vi "GUI_StagingCameras.vi"() -> ()   [LabVIEW 2013]
uses:
  shared programs/GUI_Template/GUI_master/tcp_new_data_event.ctl
  shared programs/GUI_Template/GUI_master/tcp new data cluster.ctl
  <vilib>/vision/Image Controls.llb/IMAQ Image.ctl
panel:
  in  "Target.X::9":dbl=200.0 caption="Target X" format="%#.2p"
  in  "Target.Y::9":dbl=200.0 caption="Target Y" format="%#.2p"
  in  "Target.X::8":dbl=200.0 caption="Target X" format="%#.2p"
  in  "Target.Y::8":dbl=200.0 caption="Target Y" format="%#.2p"
  in  "Target.X::7":dbl=200.0 caption="Target X" format="%#.2p"
  in  "Target.Y::7":dbl=200.0 caption="Target Y" format="%#.2p"
  in  "Target.X::6":dbl=200.0 caption="Target X" format="%#.2p"
  in  "Target.Y::6":dbl=200.0 caption="Target Y" format="%#.2p"
  in  "Target.X::5":dbl=200.0 caption="Target X" format="%#.2p"
  in  "Target.Y::5":dbl=200.0 caption="Target Y" format="%#.2p"
  in  "Target.X::4":dbl=200.0 caption="Target X" format="%#.2p"
  in  "Target.Y::4":dbl=200.0 caption="Target Y" format="%#.2p"
  in  "Target.X::3":dbl=200.0 caption="Target X" format="%#.2p"
  in  "Target.Y::3":dbl=200.0 caption="Target Y" format="%#.2p"
  in  "Target.X::2":dbl=200.0 caption="Target X" format="%#.2p"
  in  "Target.Y::2":dbl=200.0 caption="Target Y" format="%#.2p"
  in  "Target.Y::1":dbl=200.0 caption="Target Y" format="%#.2p"
  in  "Target.X::1":dbl=200.0 caption="Target X" format="%#.2p"
  in  "MaxGUIPixel::9":dbl=200.0 caption="Max GUI pixel" format="%#.2p"
  in  "MaxGUIPixel::8":dbl=200.0 caption="Max GUI pixel" format="%#.2p"
  in  "MaxGUIPixel::7":dbl=200.0 caption="Max GUI pixel" format="%#.2p"
  in  "MaxGUIPixel::6":dbl=200.0 caption="Max GUI pixel" format="%#.2p"
  in  "MaxGUIPixel::5":dbl=200.0 caption="Max GUI pixel" format="%#.2p"
  in  "MaxGUIPixel::4":dbl=200.0 caption="Max GUI pixel" format="%#.2p"
  in  "MaxGUIPixel::3":dbl=200.0 caption="Max GUI pixel" format="%#.2p"
  in  "MaxGUIPixel::2":dbl=200.0 caption="Max GUI pixel" format="%#.2p"
  in  "MaxGUIPixel::1":dbl=200.0 caption="Max GUI pixel" format="%#.2p"
  in  "Position.Axis 1::13":dbl=0.001 caption="x" step=0.003 format="%.3f"
  in  "Position.Axis 2::13":dbl=0.001 caption="y" step=0.003 format="%.3f"
  in  "Position.Axis 3::13":dbl=0.001 caption="x" step=0.001 format="%.3f"
  in  "Position.Axis 4::13":dbl=0.001 caption="y" step=0.001 format="%.3f"
  in  "GUIdevice 13":string="TREX TRA1"
  in  "Position.Axis 1::12":dbl=0.001 caption="x" step=0.003 format="%.3f"
  in  "GUIdevice 12":string="StagingTRA3"
  in  "Position.Axis 2::12":dbl=0.001 caption="y" step=0.003 format="%.3f"
  in  "Position.Axis 1::11":dbl=0.001 caption="x" step=0.003 format="%.3f"
  in  "GUIdevice 11":string="StagingTRA2"
  in  "Position.Axis 2::11":dbl=0.001 caption="y" step=0.003 format="%.3f"
  in  "Position.Axis 3::11":dbl=0.001 caption="x" step=0.0001 format="%.3f"
  in  "Position.Axis 4::11":dbl=0.001 caption="y" step=0.001 format="%.3f"
  in  "Position.Axis 5::11":dbl=0.001 caption="x" step=0.003 format="%.3f"
  in  "Position.Axis 6::11":dbl=0.001 caption="y" step=0.003 format="%.3f"
  in  "Position.Axis 6::10":dbl=0.001 caption="y" step=0.003 format="%.3f"
  in  "Position.Axis 5::10":dbl=0.001 caption="x" format="%.3f"
  in  "Position.Axis 4::10":dbl=0.001 caption="y" step=0.003 format="%.3f"
  in  "Position.Axis 3::10":dbl=0.001 caption="x" step=0.003 format="%.3f"
  in  "Position.Axis 2::10":dbl=0.001 caption="y" step=0.003 format="%.3f"
  in  "GUIdevice 10":string="StagingTRA1"
  in  "Position.Axis 1::10":dbl=0.001 caption="x" step=0.003 format="%#.3p"
  out "image::2":T1(plugin-control) caption="StagingM1Far"
  in  "exposure::2":dbl=0.001 caption="exposure" format="%#.2p"
  in  "exposure::3":dbl=0.001 caption="exposure" format="%#.2p"
  out "image::3":T1(plugin-control) caption="StagingOAP2Near"
  in  "exposure::1":dbl=0.001 caption="exposure" format="%#.2p"
  out "image::1":T1(plugin-control) caption="StagingM1Near"
  in  "GUIdevice 9":string="StagingAlignBeam2"
  in  "exposure::9":dbl=0.001 caption="exposure" format="%#.2p"
  out "image::9":T1(plugin-control) caption="StagingAlignBeam2"
  in  "exposure::8":dbl=0.001 caption="exposure" format="%#.2p"
  out "image::8":T1(plugin-control) caption="StagingOAP2Far"
  in  "exposure::7":dbl=0.001 caption="exposure" format="%#.2p"
  out "image::7":T1(plugin-control) caption="StagingOAP1Far"
  in  "GUIdevice 8":string="StagingOAP2Far"
  in  "GUIdevice 7":string="StagingOAP1Far"
  in  "GUIdevice 6":string="StagingAlignBeam1"
  in  "exposure::6":dbl=0.001 caption="exposure" format="%#.2p"
  out "image::6":T1(plugin-control) caption="StagingAlignBeam1"
  in  "exposure::5":dbl=0.001 caption="exposure" format="%#.2p"
  out "image::5":T1(plugin-control) caption="StagingOAP1Near"
  in  "exposure::4":dbl=0.001 caption="exposure" format="%#.2p"
  out "image::4":T1(plugin-control) caption="StagingM3Far"
  in  "GUIdevice 5":string="StagingOAP1Near"
  in  "GUIdevice 4":string="StagingM3Far"
  in  "GUIdevice 3":string="StagingOAP2Near"
  in  "GUIdevice 2":string="StagingM1Far"
  out "error IO 2":errorcluster
  out "tcp data event":T2
  in  "GUIdevice 1":string="StagingM1Near"
  in  "insert tag":bool=TRUE
  in  "stop":bool
  # "STAGING CAMERAS"
  # "M20"
  # "SW Mirror"
  # "M1"
  # "M3"
  # "OAP1 Mirror"
  # "BS mirror"
  # "OAP 2"
  # "M5"
  # "M4"
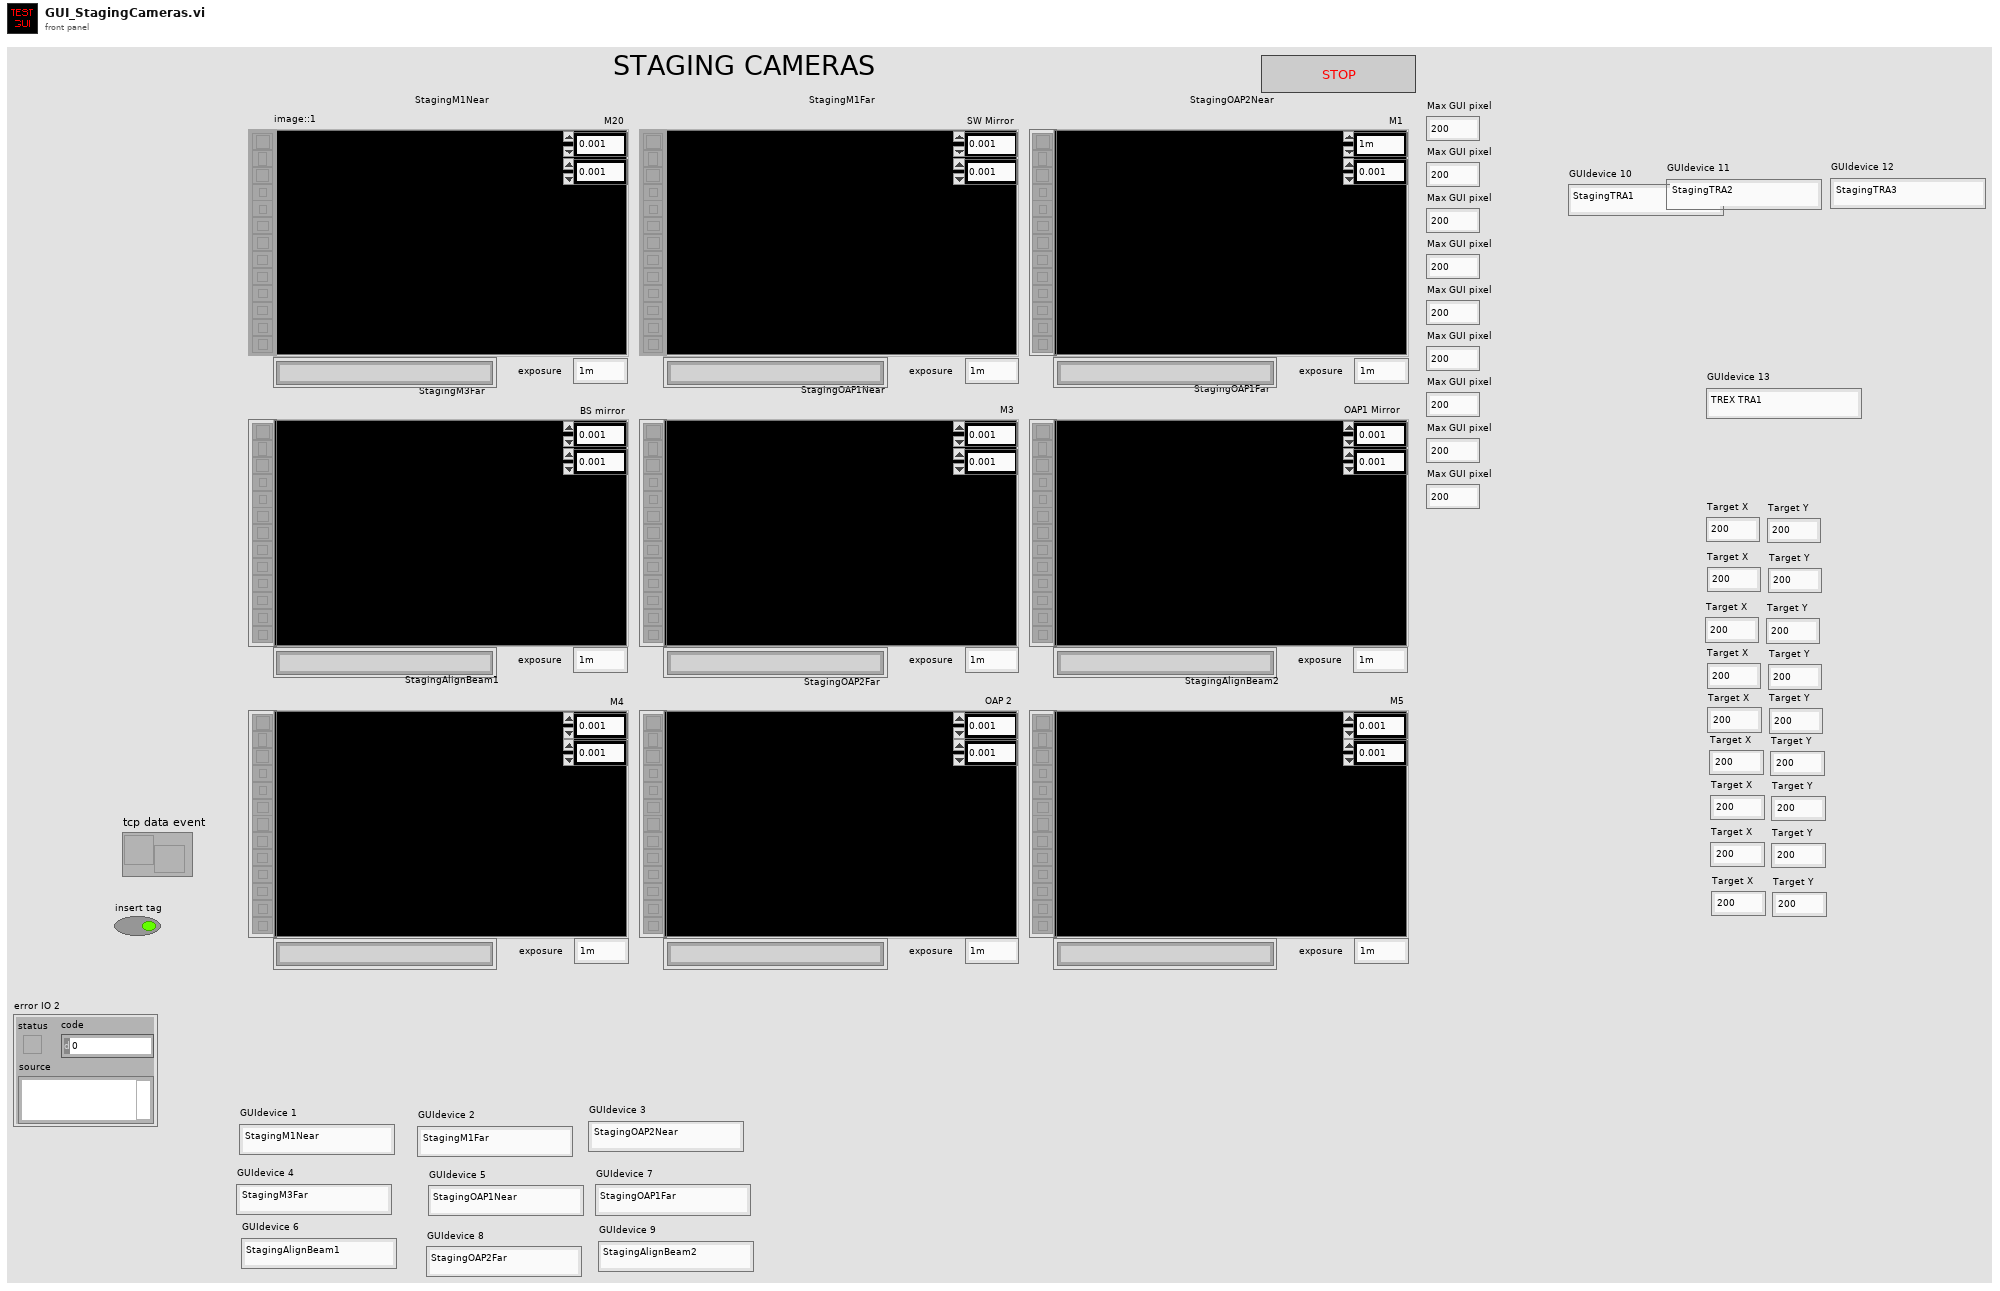
[diagram p1: front panel]
types:
  T1 = typedef "IMAQ Image.ctl" = refnum<image>
  T2 = typedef "tcp_new_data_event.ctl" = refnum<user-event>
  T3 = typedef "tcp new data cluster.ctl" = cluster{"EventEnum":enum16{"new data", "connection status update"}, "Device name":string}
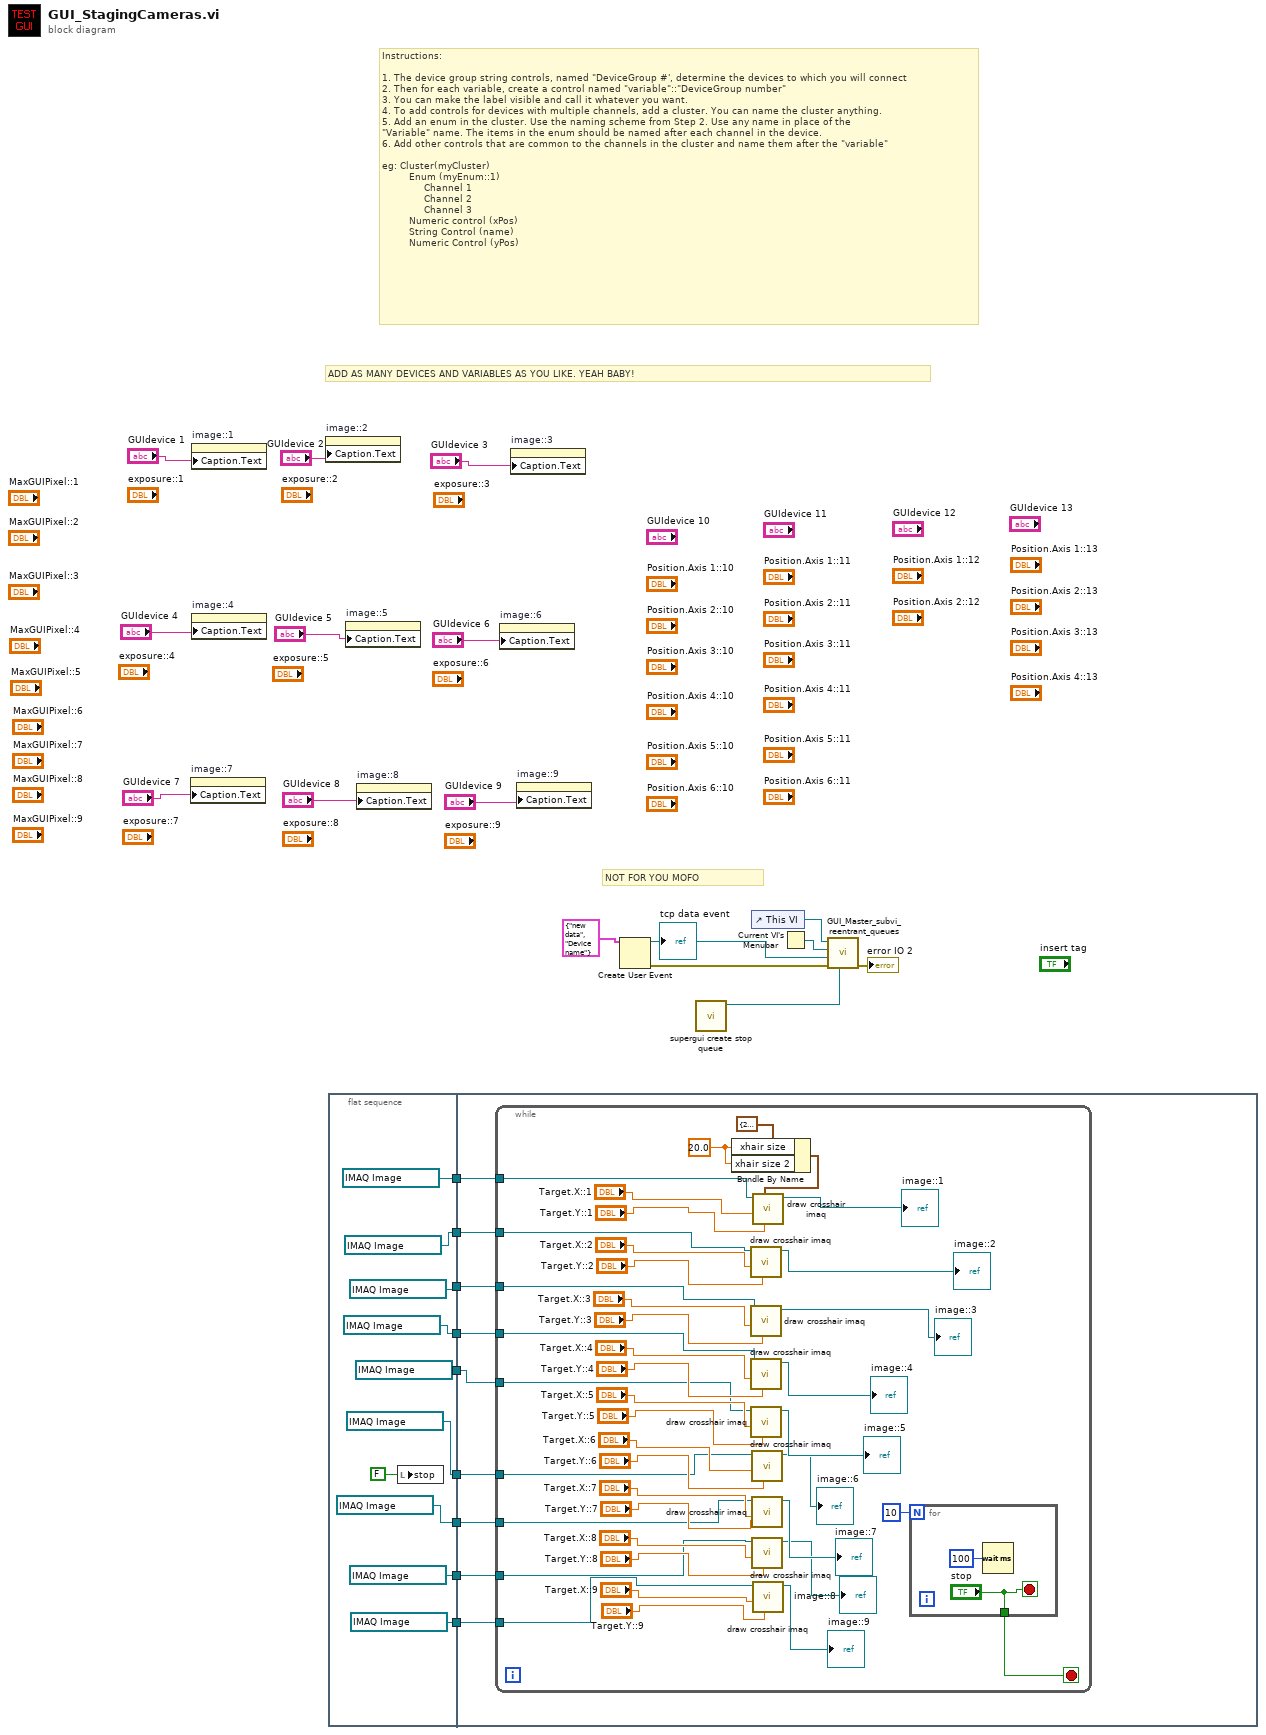
[diagram p0: block diagram]
diagram:
  # "Instructions:\n\n1. The device group string controls, named \"DeviceGroup #', determine the devices to which you will connect\n2. Then for each variable, create a control named \"variable\"::\"DeviceGroup number\"\n3. You can make the label visible and call it whatever you want.\n4. To add controls for devices with multiple channels, add a cluster. You can name the cluster anything.\n5. Add an enum in the cluster. Use the naming scheme from Step 2. Use any name in place of the \n\"Variable\" name. The items in the enum should be named after each channel in the device. \n6. Add other controls that are common to the channels in the cluster and name them after the \"variable\"\n\neg: Cluster(myCluster)\n         Enum (myEnum::1)\n              Channel 1 \n              Channel 2\n              Channel 3\n         Numeric control (xPos)\n         String Control (name)\n         Numeric Control (yPos)"
  # "ADD AS MANY DEVICES AND VARIABLES AS YOU LIKE. YEAH BABY!"
  # "NOT FOR YOU MOFO"
  n1 = property on="image::7" class="ImageControl"("Caption.Text"="GUIdevice 7") -> ()  [unwired: 2 in, 2 out]
  n2 = property on="image::1" class="ImageControl"("Caption.Text"="GUIdevice 1") -> ()  [unwired: 2 in, 2 out]
  n3 = property on="image::4" class="ImageControl"("Caption.Text"="GUIdevice 4") -> ()  [unwired: 2 in, 2 out]
  n4 = property on="image::2" class="ImageControl"("Caption.Text"="GUIdevice 2") -> ()  [unwired: 2 in, 2 out]
  n5 = flat-sequence {
    tunnel: [T1 refnum ("New Image")] -> w10
    tunnel: [T1 refnum ("New Image")] -> w9
    tunnel: [T1 refnum ("New Image")] -> w8
    tunnel: [T1 refnum ("New Image")] -> w7
    tunnel: [T1 refnum ("New Image")] -> w6
    tunnel: [T1 refnum ("New Image")] -> w5
    tunnel: [T1 refnum ("New Image")] -> w4
    tunnel: [T1 refnum ("New Image")] -> w3
    tunnel: [T1 refnum ("New Image")] -> w2
    tunnel: w10 -> [w44]
    tunnel: w9 -> [w43]
    tunnel: w8 -> [w42]
    tunnel: w7 -> [w41]
    tunnel: w6 -> [w40]
    tunnel: w5 -> [w39]
    tunnel: w4 -> [w38]
    tunnel: w3 -> [w37]
    tunnel: w2 -> [w36]
    frame #0 {
      n6 = local write "stop"(FALSE ("stop")) -> ()
    }
    frame #1 {
      n7 = while {
        tunnel: w44 -> [w67]
        tunnel: w43 -> [w63]
        tunnel: w42 -> [w60]
        tunnel: w41 -> [w58]
        tunnel: w40 -> [w57]
        tunnel: w39 -> [w55]
        tunnel: w38 -> [w53]
        tunnel: w37 -> [w50]
        tunnel: w36 -> [w48]
        stop <- w64 stop-if-true
        w46 = 20.0 ("size")
        n8 = Bundle By Name(cluster=cluster{"xhair size":dbl, "xhair size 2":dbl} {"xhair size"=20.0, "xhair size 2"=20.0} ("size"), "xhair size"=w46, "xhair size 2"=w46) -> (w45:cluster{"xhair size":dbl, "xhair size 2":dbl})
        n9 = call "draw crosshair imaq.vi"("Target.Y"="Target.Y::2", "Target.X"="Target.X::2", "image in"=w63) -> ("image out"=→"image::2":T1)  [unwired: 7 in, 1 out]
        n10 = call "draw crosshair imaq.vi"("Target.Y"="Target.Y::3", "Target.X"="Target.X::3", "image in"=w60) -> ("image out"=→"image::3":T1)  [unwired: 7 in, 1 out]
        n11 = call "draw crosshair imaq.vi"("Target.Y"="Target.Y::4", "Target.X"="Target.X::4", "image in"=w58) -> ("image out"=→"image::4":T1)  [unwired: 7 in, 1 out]
        n12 = call "draw crosshair imaq.vi"("Target.Y"="Target.Y::5", "Target.X"="Target.X::5", "image in"=w57) -> ("image out"=→"image::5":T1)  [unwired: 7 in, 1 out]
        n13 = call "draw crosshair imaq.vi"("Target.Y"="Target.Y::6", "Target.X"="Target.X::6", "image in"=w55) -> ("image out"=→"image::6":T1)  [unwired: 7 in, 1 out]
        n14 = call "draw crosshair imaq.vi"("Target.Y"="Target.Y::7", "Target.X"="Target.X::7", "image in"=w53) -> ("image out"=→"image::7":T1)  [unwired: 7 in, 1 out]
        n15 = call "draw crosshair imaq.vi"("Target.Y"="Target.Y::8", "Target.X"="Target.X::8", "image in"=w50) -> ("image out"=→"image::8":T1)  [unwired: 7 in, 1 out]
        n16 = call "draw crosshair imaq.vi"("Target.Y"="Target.Y::1", "size"=w45, "Target.X"="Target.X::1", "image in"=w67) -> ("image out"=→"image::1":T1)  [unwired: 6 in, 1 out]
        n17 = call "draw crosshair imaq.vi"("Target.Y"="Target.Y::9", "Target.X"="Target.X::9", "image in"=w48) -> ("image out"=→"image::9":T1)  [unwired: 7 in, 1 out]
        n18 = for {
          N: 10 -> [_]
          tunnel: ["stop"] -> w64
          stop <- "stop" stop-if-true
          n19 = Wait (ms)(milliseconds to wait=u32 100) -> ()  [unwired: 1 out]
        }
      }
    }
  }
  n20 = property on="image::5" class="ImageControl"("Caption.Text"="GUIdevice 5") -> ()  [unwired: 2 in, 2 out]
  n21 = property on="image::8" class="ImageControl"("Caption.Text"="GUIdevice 8") -> ()  [unwired: 2 in, 2 out]
  n22 = property on="image::6" class="ImageControl"("Caption.Text"="GUIdevice 6") -> ()  [unwired: 2 in, 2 out]
  n23 = property on="image::3" class="ImageControl"("Caption.Text"="GUIdevice 3") -> ()  [unwired: 2 in, 2 out]
  n24 = property on="image::9" class="ImageControl"("Caption.Text"="GUIdevice 9") -> ()  [unwired: 2 in, 2 out]
  n25 = Create User Event(user event datatype=T3 {"EventEnum"=enum."new data", "Device name"="Device name"} ("New Event")) -> (user event=w20:refnum<user-event>, error out=w21:errorcluster)  [unwired: 1 in]
  "tcp data event" <- w20
  n26 = call "supergui create stop queue.vi"() -> ("STOP Queue out"=w1:refnum<queue>)  [unwired: 11 in]
  n27 = control-ref of="This VI"() -> (w24:refnum<vi>)
  n28 = Current VI's Menubar() -> (w23:refnum<k9>)
  n29 = call "GUI_Master_subvi_reentrant_queues.vi"("STOP Queue in"=w1, "error in (no error)"=w21, "tcp data event"=w20, "Caller menu reference"=w23, "Caller VI ref"=w24) -> ("error out"=→"error IO 2":errorcluster)  [unwired: 6 in]
